vi "FPGA_target_set_output.vi"(3 "tick_count_in":u32, 4 "data_in":T1, 6 "new_data_in":T1, 7 "set_outputs":bool=TRUE, 9 "C0_data":T2, 11 "C1_data":T2) -> (17 "tick_count_out":u32, 18 "data_out":T1)   [LabVIEW 2014]
doc: "writes a 64 bit pattern to the output lines"
uses:
  FPGA_32BitPattern_data_type.ctl
  FPGA_cmd_data_type.ctl
  <vilib>/rvi/eio/common/nirviEmuTemplateMethod_errors.vi
  <vilib>/eio/EIONode/EIONode.xnode
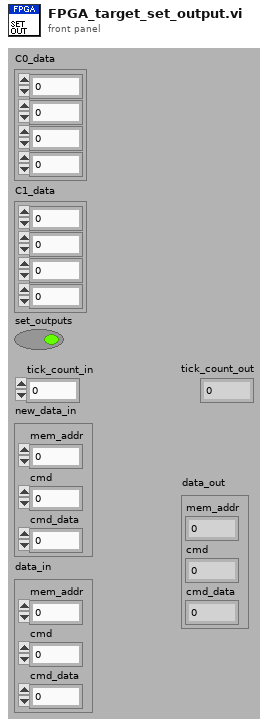
[diagram p1: front panel]
types:
  T1 = typedef "FPGA_cmd_data_type.ctl" = cluster{"mem_addr":u32, "cmd":u8, "cmd_data":u32}
  T2 = typedef "FPGA_32BitPattern_data_type.ctl" = cluster{"port0":u8, "port1":u8, "port2":u8, "port3":u8}
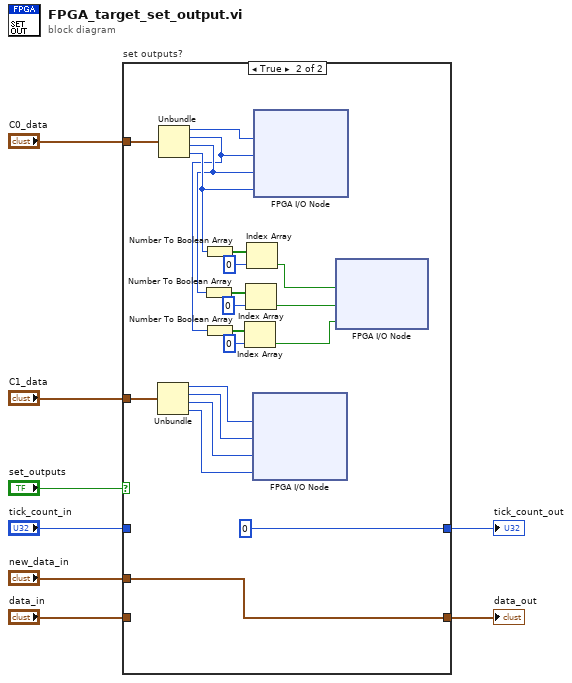
[diagram p0: block diagram]
diagram:
  n1 = case "set outputs?" shown="True" "set_outputs" {
    tunnel: [w10 u32 0] -> w8
    tunnel: "tick_count_in" -> [w10 _]
    tunnel: "C0_data" -> [_ w31]
    tunnel: "C1_data" -> [_ w25]
    tunnel: "new_data_in" -> [_ w23]
    tunnel: [w9 w23] -> w2
    tunnel: "data_in" -> [w9 _]
    frame False {
    }
    frame True {
      n2 = Unbundle(w25) -> ("port0"=w26:u8, "port1"=w27:u8, "port2"=w28:u8, "port3"=w29:u8)
      n3 = Unbundle(w31) -> ("port0"=w30:u8, "port1"=w12:u8, "port2"=w16:u8, "port3"=w22:u8)
      n4 = Number To Boolean Array(number=w16) -> (Boolean array=w18:bool[])
      n5 = Number To Boolean Array(number=w22) -> (Boolean array=w21:bool[])
      n6 = Number To Boolean Array(number=w12) -> (Boolean array=w14:bool[])
      n7 = Index Array(array=w14, index=0) -> (element=w11:bool)
      n8 = Index Array(array=w18, index=0) -> (element=w15:bool)
      n9 = Index Array(array=w21, index=0) -> (element=w19:bool)
      n10 = xnode ("FPGA I/O Node")("DO_56-63"=w26, "DO_48-55"=w27, "DO_40-47"=w28, "DO_32-39"=w29) -> ()  [unwired: 4 in, 4 out]
      n11 = xnode ("FPGA I/O Node")("DO_24-31"=w30, "DO_16-23"=w12, "DO_08-15"=w16, "DO_00-07"=w22) -> ()  [unwired: 4 in, 4 out]
      n12 = xnode "FPGA I/O Node"("PXI_Trig0"=w19, "PXI_Trig1"=w15, "PXI_Trig2"=w11) -> ()  [unwired: 3 in, 3 out]
    }
  }
  "tick_count_out" <- w8
  "data_out" <- w2
